vi "Set_shutdown_HV.vi"() -> ()   [LabVIEW 2012]
uses:
  hv cluster control.ctl
  <vilib>/Platform/TimedLoop/XDataNode/timing_clust.ctl
  <vilib>/Platform/TimedLoop/XDataNode/nitl_modes.ctl
  <vilib>/Platform/TimedLoop/XDataNode/wakeup.ctl
  <vilib>/Platform/TimedLoop/XDataNode/XDataNode.xnode
  CAEN/labview/CAENHVWrapper/CAENHVWrapper.lvlib
  <vilib>/Platform/TimedLoop/XDataNode/XDNodeRunTimeDep.lvlib
panel:
  out "Current(uA)":sgl[](array[numeric])
  out "HV (V)":sgl[](array[numeric])
  in  "stop":bool
  in  "Set the HVs":bool=TRUE
  in  "HV Power On/Off":bool[](array[boolean])=[TRUE, TRUE, TRUE, TRUE, TRUE, TRUE, TRUE, TRUE]
  in  "HV Tolerance (%)":dbl=1.0
  in  "Set Voltage":string[](array[string])=["620", "510", "680", "700", "990", "670", "690", "760"]
  out "handle":i32
  in  "IP adress HV2":string="1_0_0"
  in  "IP adress HV1":string="0_0_0"
  in  "HV Cluster":T1={"HV Power On/Off"=[TRUE, TRUE], "Set Voltage(V)"=["0", "0", "0", "0", "0", "0", "0", "0"], "HV Tolerance (%)"=1.0, "Current(uA)"=[]}
  # "Turn off HVs"
  # "This VI is needed to set the\nvoltages of the HV and turning channels on or off. The settings are directly fed with 'shared variables'\nto the Host program."
  # "Channel 0"
  # "The IP adress of the High Voltages depends on how you connected the two CAEN HVs, you can test which one  is which by first turning on the first 4 \nchannels and see which HV is turned on, this should then be HV1.\n\nWhen you want to shut down the HVs, just turn the switch to 'Turn off HVs' and run the VI."
  # "Channel 1"
  # "Channel 2"
  # "Channel 3"
  # "Channel 4"
  # "Channel 5"
  # "Channel 6"
  # "Channel 7"
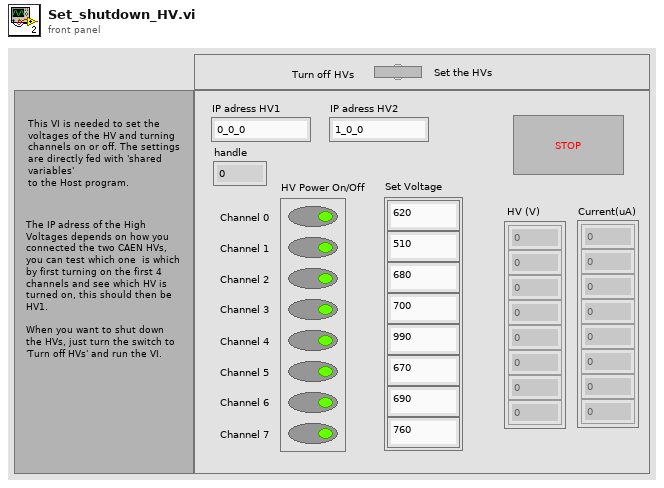
[diagram p1: front panel]
types:
  T1 = typedef "hv cluster control.ctl" = cluster{"HV Power On/Off":bool[], "Set Voltage(V)":string[], "HV Tolerance (%)":dbl, "Current(uA)":dbl[]}
  T2 = typedef "XDNodeRunTimeDep.lvlib/timing_clust.ctl" = cluster{"Expected End [f-1]":u64, "Actual End [f-1]":u64, "Finished Late? [f-1]":bool, "Expected End [i-1]":u64, "Actual End [i-1]":u64, "Finished Late? [i-1]":bool, "Expected Start [i]":u64, "Actual Start [i]":u64, "Expected Start [f]":u64, "Actual Start [f]":u64, "Source Name":string, "Structure Name":string, "Period":i64, "Deadline":i64, "Offset":i64, "Start":i64, "Priority":i32, "Timeout":i32, "Mode":T3, "Wakeup Reason":T4, "Error":errorcluster, "Source Type":string, "Secondary Source Type":string, "Global End Time":u64, "Global Start Time":u64, "Frame Duration":u64, "Iteration Duration":u64, "Assigned CPU":i32, "I/O Scan Engine Mode":u32}
  T3 = typedef "XDNodeRunTimeDep.lvlib/nitl_modes.ctl" = enum32{"No Change", "Process missed periods, maintain original phase", "Discard missed periods, maintain original phase", "Process missed periods, ignore original phase", "Discard missed periods, ignore original phase"}
  T4 = typedef "XDNodeRunTimeDep.lvlib/wakeup.ctl" = enum32{"Normal", "Aborted", "Asynchronous wakeup", "Timing source error", "Timed loop error", "Timeout"}
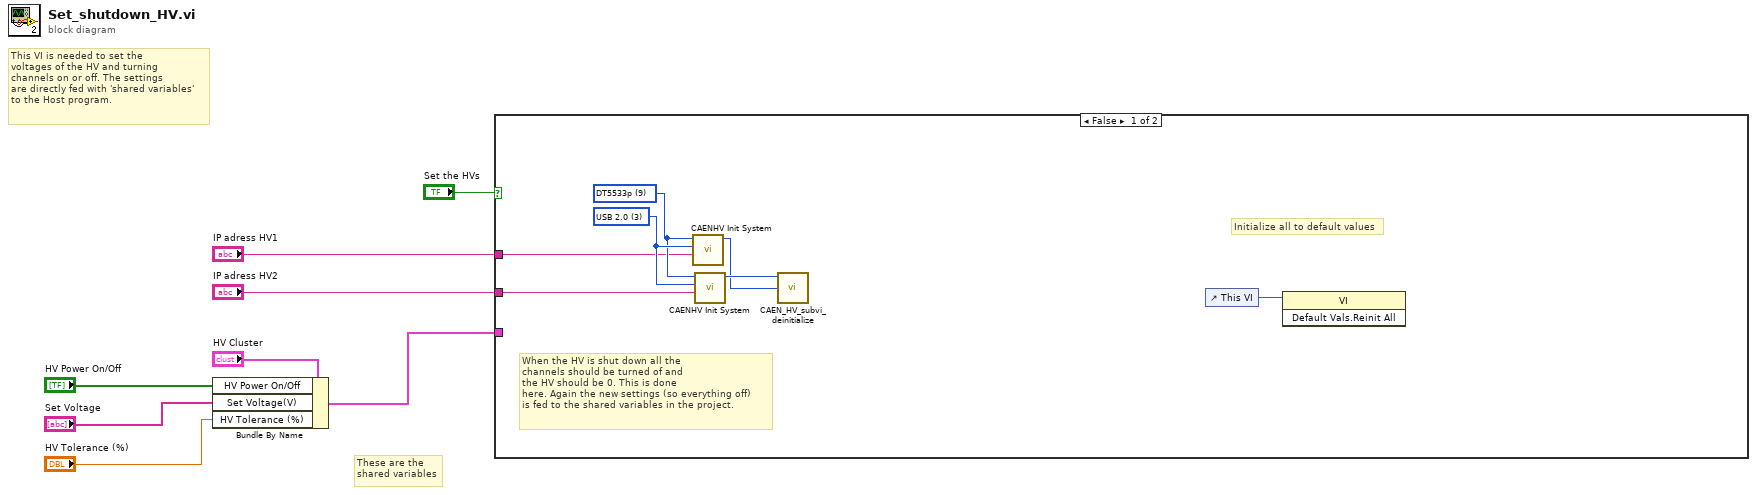
[diagram p0: block diagram]
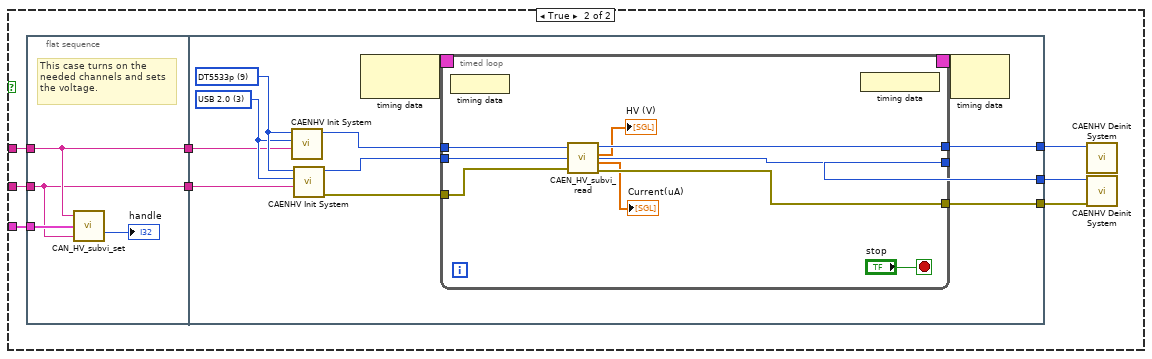
[diagram p2: hidden frame]
diagram:
  # "These are the\nshared variables"
  # "This VI is needed to set the\nvoltages of the HV and turning \nchannels on or off. The settings \nare directly fed with 'shared variables'\nto the Host program."
  n1 = Bundle By Name(cluster="HV Cluster", "HV Power On/Off"="HV Power On/Off", "Set Voltage(V)"="Set Voltage", "HV Tolerance (%)"="HV Tolerance (%)") -> (w6:T1)
  n2 = case shown="False" "Set the HVs" {
    tunnel: "IP adress HV1" -> [w11 w22]
    tunnel: "IP adress HV2" -> [w10 w21]
    tunnel: w6 -> [_ w23]
    frame False {
      w15 = 3 items=["TCP/IP"=0, "HS CAENET"=2, "USB 2.0"=3, "CONET Optical Link"=4, "USB VCP"=5] ("LinkType")
      w14 = u32 9 items=["SY1527", "SY2527", "SY4527", "SY5527", "N568", "V65XX", "N1470", "V8100", "", "DT5533p"] ("system")
      # "When the HV is shut down all the\nchannels should be turned of and \nthe HV should be 0. This is done \nhere. Again the new settings (so everything off)\nis fed to the shared variables in the project."
      # "Initialize all to default values"
      n3 = call "CAENHV Init System.vi"("Arg"=w11, "LinkType"=w15, "system"=w14) -> ("handle"=w12:i32)  [unwired: 7 in, 1 out]
      n4 = call "CAENHV Init System.vi"("Arg"=w10, "LinkType"=w15, "system"=w14) -> ("handle"=w13:i32)  [unwired: 7 in, 1 out]
      n5 = call "CAEN_HV_subvi_deinitialize.vi"("Handle 2"=w13, "Handle 1"=w12) -> ()  [unwired: 1 in, 1 out]
      n6 = control-ref of="This VI"() -> (w9:refnum<vi>)
      n7 = invoke class="VI" method="Default Vals.Reinit All"(reference=w9) -> ()  [unwired: 2 in, 3 out]
    }
    frame True {
      n8 = flat-sequence {
        tunnel: w23 -> [w26]
        tunnel: w22 -> [w25]
        tunnel: w21 -> [w24]
        tunnel: [w25] -> w20
        tunnel: [w24] -> w19
        tunnel: w20 -> [w33]
        tunnel: w19 -> [w32]
        tunnel: [w30] -> w18
        tunnel: [w29] -> w17
        tunnel: [w28] -> w16
        frame #0 {
          # "This case turns on the\nneeded channels and sets\nthe voltage."
          n9 = call "CAN_HV_subvi_set.vi"("IP adress HV2"=w24, "HV Cluster"=w26, "IP adress HV1"=w25) -> ("handle"=→"handle":i32)  [unwired: 1 out]
        }
        frame #1 {
          w34 = 3 items=["TCP/IP"=0, "HS CAENET"=2, "USB 2.0"=3, "CONET Optical Link"=4, "USB VCP"=5] ("LinkType")
          w35 = u32 9 items=["SY1527", "SY2527", "SY4527", "SY5527", "N568", "V65XX", "N1470", "V8100", "", "DT5533p"] ("system")
          n10 = call "CAENHV Init System.vi"("Arg"=w33, "LinkType"=w34, "system"=w35) -> ("handle"=w36:i32)  [unwired: 7 in, 1 out]
          n11 = call "CAENHV Init System.vi"("Arg"=w32, "LinkType"=w34, "system"=w35) -> ("error out"=w31:errorcluster, "handle"=w37:i32)  [unwired: 7 in]
          n12 = node-c288() -> (w39:T2)  [unwired: 1 in]
          n13 = timed-loop {
            timing: w39 -> [_]
            timing-out: [_] -> w38
            tunnel: w36 -> [w47]
            tunnel: w37 -> [w46]
            tunnel: w31 -> [w45]
            tunnel: [w44] -> w30
            tunnel: [w43] -> w29
            tunnel: [w42] -> w28
            stop <- "stop" stop-if-true
            n14 = node-c288() -> ()  [unwired: 1 in]
            n15 = call "CAEN_HV_subvi_read.vi"("handle HV1"=w47, "handle HV2"=w46, "error in (no error)"=w45) -> ("handle HV1 out"=w44:i32, "HV"=→"HV (V)":sgl[], "Current"=→"Current(uA)":sgl[], "error out"=w42:errorcluster, "handle HV2 out"=w43:i32)
            n16 = node-c288() -> ()  [unwired: 1 out]
          }
          n17 = node-c288(w38) -> ()  [unwired: 1 out]
        }
      }
      n18 = call "CAENHV Deinit System.vi"("handle"=w18) -> ()  [unwired: 10 in, 1 out]
      n19 = call "CAENHV Deinit System.vi"("error in (no error)"=w16, "handle"=w17) -> ()  [unwired: 9 in, 1 out]
    }
  }
